vi "Read_Data_Error.vi"(7 "path":path, 8 "error in (no error)":errorcluster, 10 "file size (in samples)":dbl format="%#_6f", 11 "runtime":u32) -> (0 "error out":errorcluster)   [LabVIEW 2016]
panel:
  in  "file size (in bytes)":dbl format="%#_6f"
  in  "bytes per sample":dbl format="%#_6f"
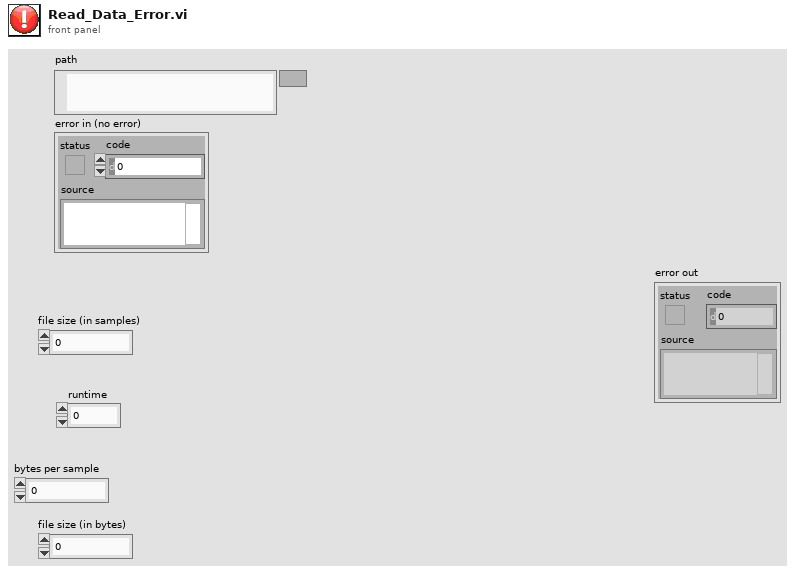
[diagram p1: front panel]
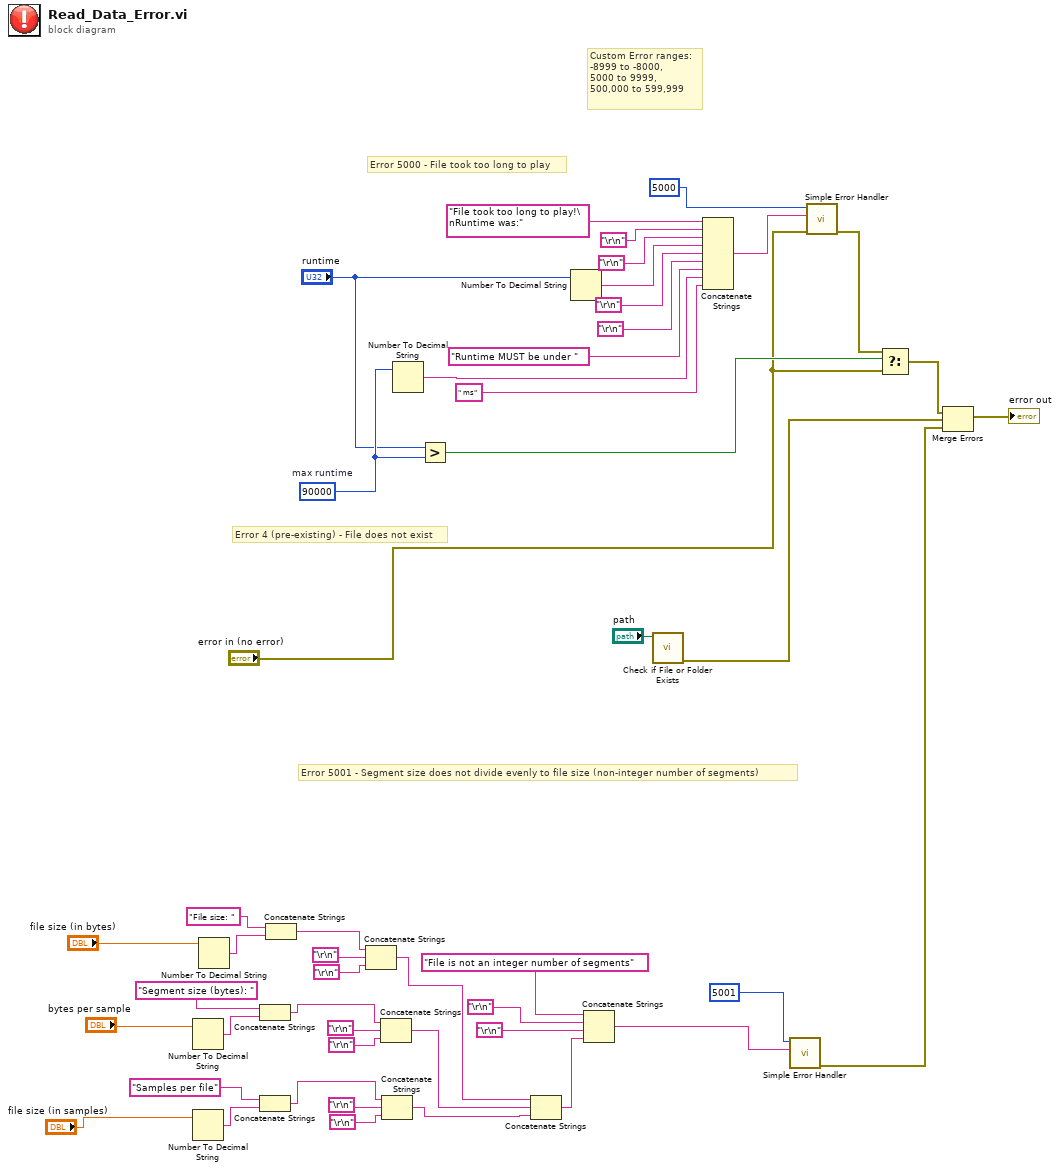
[diagram p0: block diagram]
diagram:
  w32 = 90000  # max runtime
  # "Error 5001 - Segment size does not divide evenly to file size (non-integer number of segments)"
  # "Error 4 (pre-existing) - File does not exist"
  # "Error 5000 - File took too long to play"
  # "Custom Error ranges:\n-8999 to -8000, \n5000 to 9999,\n500,000 to 599,999"
  n1 = Number To Decimal String(number="bytes per sample") -> (decimal integer string=w24:string)  [unwired: 1 in]
  n2 = Number To Decimal String(number="file size (in samples)") -> (decimal integer string=w22:string)  [unwired: 1 in]
  n3 = Number To Decimal String(number="file size (in bytes)") -> (decimal integer string=w26:string)  [unwired: 1 in]
  n4 = Concatenate Strings("Segment size (bytes): ", w24) -> (w7:string)
  n5 = Concatenate Strings("Samples per file", w22) -> (w8:string)
  n6 = Concatenate Strings("File size: ", w26) -> (w17:string)
  n7 = Concatenate Strings(w17, "\r\n", "\r\n") -> (w10:string)
  n8 = Concatenate Strings(w7, "\r\n", "\r\n") -> (w9:string)
  n9 = Concatenate Strings(w8, "\r\n", "\r\n") -> (w1:string)
  n10 = Number To Decimal String(number=w32) -> (decimal integer string=w33:string)  [unwired: 1 in]
  n11 = Greater?(x="runtime", y=w32) -> (0:w31:bool)
  n12 = Concatenate Strings(w10, w9, w1) -> (w6:string)
  n13 = Number To Decimal String(number="runtime") -> (decimal integer string=w40:string)  [unwired: 1 in]
  n14 = Concatenate Strings("File is not an integer number of segments", "\r\n", "\r\n", w6) -> (w2:string)
  n15 = call <vilib>:"Check if File or Folder Exists.vi"("path"="path") -> ("error out"=w38:errorcluster)  [unwired: 8 in, 2 out]
  n16 = Concatenate Strings("File took too long to play!\nRuntime was:", "\r\n", "\r\n", w40, "\r\n", "\r\n", "Runtime MUST be under ", w33, " ms") -> (w48:string)
  n17 = call <vilib>:"Simple Error Handler.vi"("error code (no error:0)"=5001, "error source (\" \")"=w2) -> ("error out"=w5:errorcluster)  [unwired: 3 in, 4 out]
  n18 = call <vilib>:"Simple Error Handler.vi"("error code (no error:0)"=5000, "error source (\" \")"=w48, "error in (no error)"="error in (no error)") -> ("error out"=w35:errorcluster)  [unwired: 2 in, 4 out]
  n19 = Select(t=w35, s=w31, f="error in (no error)") -> (s? t:f=w36:errorcluster)
  n20 = Merge Errors(w36, w38, w5) -> (→"error out":errorcluster)
